vi "Read commandName.vi"(8 "error in (no error)":errorcluster, 11 "Enable in":refnum<class "enable.lvclass">) -> (0 "error out":errorcluster, 2 "CommandValue":T1, 3 "Enable out":refnum<class "enable.lvclass">)   [LabVIEW 2016, in "Commands.lvlib" / "enable.lvclass"]
uses:
  enable.lvclass
  Typedefs/CommandValue.ctl
  Typedefs/EXATypedefs.lvlib
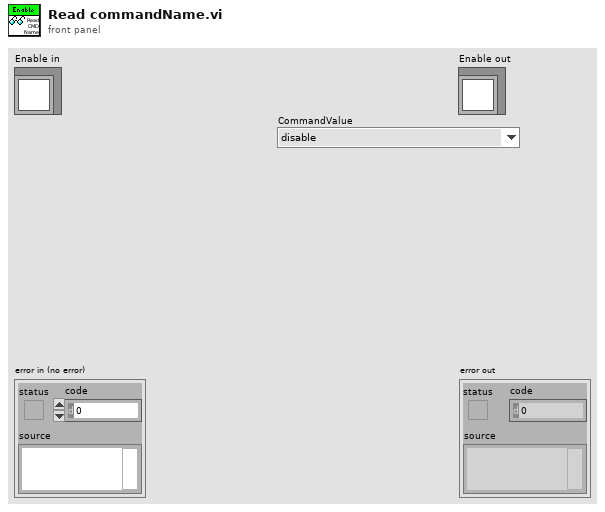
[diagram p1: front panel]
types:
  T1 = typedef "EXATypedefs.lvlib/CommandValue.ctl" = enum16{"disable", "enable", "exit", "GoToStandby", "OnHeartbeat", "OnIncomingMessagingError", "OnInterrupt", "start", "captureSpectImage", "setSpectTempSetpoint", "stopImageCapture"}
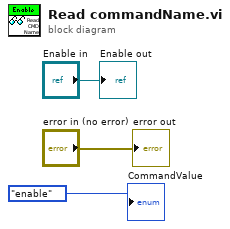
[diagram p0: block diagram]
diagram:
  "error out" <- "error in (no error)"
  "Enable out" <- "Enable in"
  "CommandValue" <- CommandValue."enable" ("CommandValue")
